vi "ep_Check Fundamental Phase Parameters.vi"(4 "actual ranges [%]":dbl[](array[numeric]), 6 "ranges to calibrate [%]":dbl[](array[numeric]), 8 "error in (no error)":errorcluster, 10 "phase delays [deg]":dbl[][](array[numeric]), 11 "one-cycle fundamental vectors in":T2(array[cluster])) -> (0 "error out":errorcluster)   [LabVIEW 2014, in "NI_EP_Power Quality.lvlib"]
uses:
  <vilib>/addons/Electrical Power/PQ/Common/Controls/ep_AI Data Channel.ctl
  <vilib>/addons/Electrical Power/PQ/NI_EP_Power Quality.lvlib
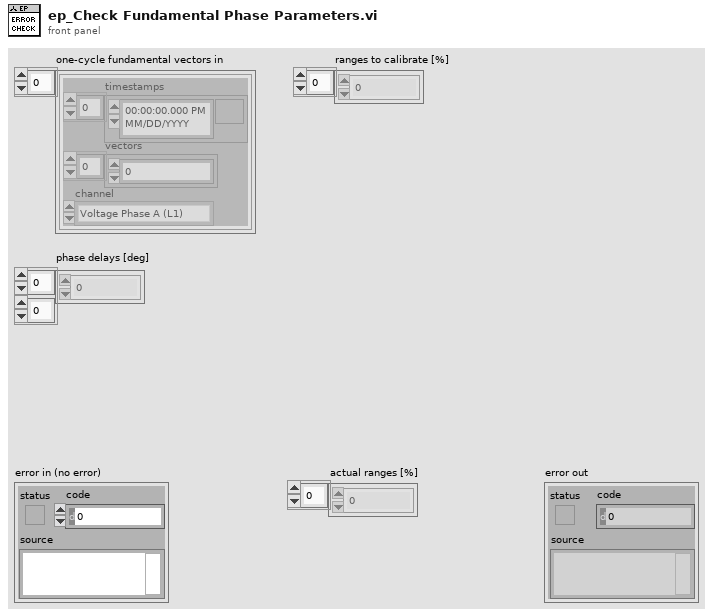
[diagram p1: front panel]
types:
  T1 = typedef "NI_EP_Power Quality.lvlib/ep_AI Data Channel.ctl" = enum16{"Voltage Phase A (L1)", "Voltage Phase B (L2)", "Voltage Phase C (L3)", "Voltage Phase N (Neutral)", "Current Phase A (L1)", "Current Phase B (L2)", "Current Phase C (L3)", "Current Phase N (Neutral)"}
  T2 = cluster{"timestamps":timestamp[], "vectors":cdb[], "channel":T1}[]
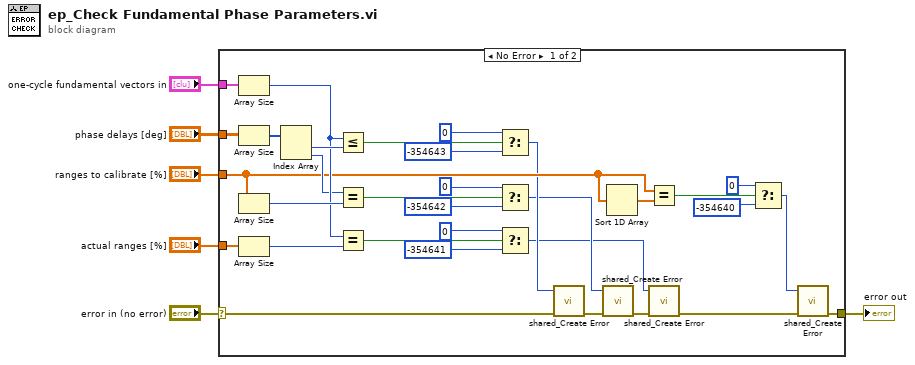
[diagram p0: block diagram]
diagram:
  n1 = case shown="No Error" "error in (no error)" {
    selector: "error in (no error)" -> [w7 w39]
    tunnel: "one-cycle fundamental vectors in" -> [w27 _]
    tunnel: "phase delays [deg]" -> [w26 _]
    tunnel: "ranges to calibrate [%]" -> [w25 _]
    tunnel: "actual ranges [%]" -> [w24 _]
    tunnel: [w8 w39] -> w2
    frame No Error {
      n2 = Array Size(array=w27) -> (size(s)=w34:i32)
      n3 = Array Size(array=w26) -> (size(s)=w36:i32[])
      n4 = Array Size(array=w25) -> (size(s)=w37:i32)
      n5 = Array Size(array=w24) -> (size(s)=w38:i32)
      n6 = Index Array(array=w36) -> (element #1=w35:i32, element #2=w33:i32)  [unwired: 2 in]
      n7 = Less Or Equal?(x=w34, y=w35) -> (x <= y?=w28:bool)
      n8 = Equal?(x=w33, y=w37) -> (x = y?=w29:bool)
      n9 = Equal?(x=w34, y=w38) -> (x = y?=w30:bool)
      n10 = Select(t=0 ("error code (0)"), s=w28, f=-354643 ("error code (0)")) -> (s? t:f=w19:i32)
      n11 = Select(t=0 ("error code (0)"), s=w29, f=-354642 ("error code (0)")) -> (s? t:f=w16:i32)
      n12 = Select(t=0 ("error code (0)"), s=w30, f=-354641 ("error code (0)")) -> (s? t:f=w13:i32)
      n13 = call <vilib>:"shared_Create Error.vi"("error in (no error)"=w7, "error code (0)"=w19) -> ("error out"=w17:errorcluster)  [unwired: 9 in]
      n14 = call <vilib>:"shared_Create Error.vi"("error in (no error)"=w17, "error code (0)"=w16) -> ("error out"=w15:errorcluster)  [unwired: 9 in]
      n15 = Sort 1D Array(array=w25) -> (sorted array=w32:dbl[])
      n16 = Equal?(x=w25, y=w32) -> (x = y?=w31:bool)
      n17 = call <vilib>:"shared_Create Error.vi"("error in (no error)"=w15, "error code (0)"=w13) -> ("error out"=w9:errorcluster)  [unwired: 9 in]
      n18 = Select(t=0 ("error code (0)"), s=w31, f=-354640 ("error code (0)")) -> (s? t:f=w10:i32)
      n19 = call <vilib>:"shared_Create Error.vi"("error in (no error)"=w9, "error code (0)"=w10) -> ("error out"=w8:errorcluster)  [unwired: 9 in]
    }
    frame Error {
    }
  }
  "error out" <- w2
